vi "Get Twiddle Factors from BRAM.vi"(1 "Address Type":T1, 2 "Reset?":bool, 7 "Input Data Valid":bool) -> (6 "cosine":fxp<+/-,18,1> format="%.18g", 8 "sine":fxp<+/-,18,1> format="%.18g", 10 "Output Valid":bool, 14 "phase_out":fxp<+/-,14,1> format="%.14g")   [LabVIEW 2011]
doc: "This VI has delay of 7 Ticks"
uses:
  <vilib>/rvi/XilinxIP/XIPIN_XNode/niFpgaXIPIN.xnode
  <vilib>/rvi/FXPMathLib/basic elements/FxpDiscreteDelay/XNode/nifxpmath_DiscreteDelay.xnode
  <userlib>/FPGA Library/Code Development/Signal Processing/FFT Block/Twiddle Factor/LUT/Get Twiddle Factors from BRAM/SinCosLUT/SinCosLUT_B722A32F442EF2B1197D819CB4159066.dll
  <vilib>/rvi/IPIntegrationNode/IPINode_Xnode/niFpgaIPINode.xnode
  <userlib>/FPGA Library/Code Development/Signal Processing/FFT Block/Twiddle Factor/Address Generation/Twiddle Address FXP Type.ctl
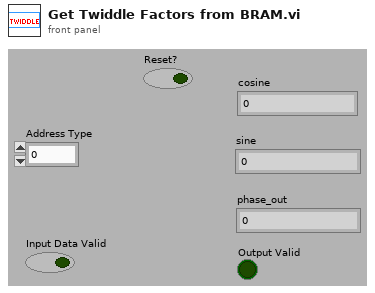
[diagram p1: front panel]
types:
  T1 = typedef "Twiddle Address FXP Type.ctl" = fxp<+,9,9>
  T2 = typedef "BRAM Phase FXP Type.ctl" = fxp<+/-,14,1>
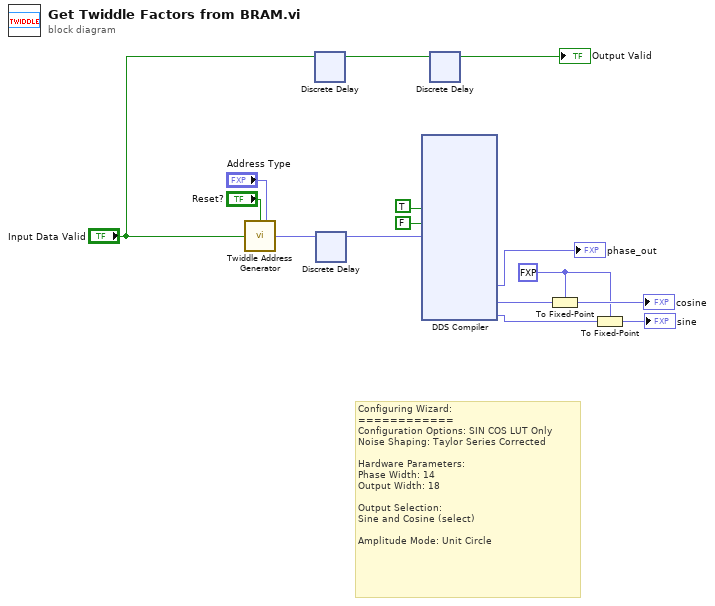
[diagram p0: block diagram]
diagram:
  w3 = fxp<+/-,18,1> 0.0
  # "Configuring Wizard:\n============\nConfiguration Options: SIN COS LUT Only\nNoise Shaping: Taylor Series Corrected\n\nHardware Parameters:\nPhase Width: 14\nOutput Width: 18\n\nOutput Selection:\nSine and Cosine (select)\n\nAmplitude Mode: Unit Circle"
  n1 = call <userlib>:"Twiddle Address Generator.vi"("Reset?"="Reset?", "Address Type"="Address Type", "Increment?"="Input Data Valid") -> ("Twiddle Address"=w9:T2)  [unwired: 12 in]
  n2 = xnode "Discrete Delay"("D"="Input Data Valid") -> ("Q"=w1:bool)
  n3 = xnode "Discrete Delay"("D"=w9) -> ("Q"=w2:fxp<+/-,14,1>)
  n4 = xnode ("DDS Compiler")("ce"=TRUE, "sclr"=FALSE, "phase_in"=w2) -> ("phase_out"=→"phase_out":fxp<+/-,14,1>, "cosine"=w7:fxp<+/-,18,2>, "sine"=w6:fxp<+/-,18,2>)  [unwired: 2 out]
  n5 = xnode "Discrete Delay"("D"=w1) -> ("Q"=→"Output Valid":bool)
  n6 = To Fixed-Point(fixed-point type=w3, number=w7) -> (fixed-point=→"cosine":fxp<+/-,18,1>)
  n7 = To Fixed-Point(fixed-point type=w3, number=w6) -> (fixed-point=→"sine":fxp<+/-,18,1>)
